vi "vapor_density.vi"(0 "Vapor Temp [C]":dbl) -> (1 "Vapor Density[g/cm3]":dbl, 2 "formula":string=" 0.218237*exp(0.0354887*T) ")   [LabVIEW 2017]
uses:
  <vilib>/gmath/NI_Gmath.lvlib
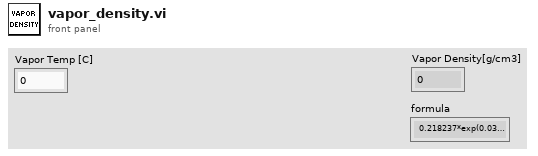
[diagram p1: front panel]
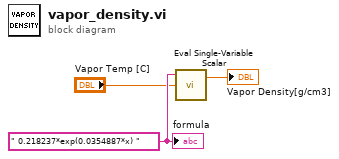
[diagram p0: block diagram]
diagram:
  w3 = " 0.218237*exp(0.0354887*x) " ("formula")
  n1 = call <vilib>:"Eval Single-Variable Scalar.vi"("x value"="Vapor Temp [C]", "formula"=w3) -> ("y value"=→"Vapor Density[g/cm3]":dbl)  [unwired: 1 in, 1 out]
  "formula" <- w3
